vi "FGV_Id_Iq_ES.vi"(6 "Buffer Size":i32=10000, 7 "Command":T1, 8 "error in (no error)":errorcluster, 10 "Iq":sgl, 11 "Id":sgl) -> (0 "error out":errorcluster, 3 "Buffer":sgl[][](array[numeric]), 5 "Buffer Index":i32)   [LabVIEW 2015]
uses:
  Data_Queue_Command.ctl
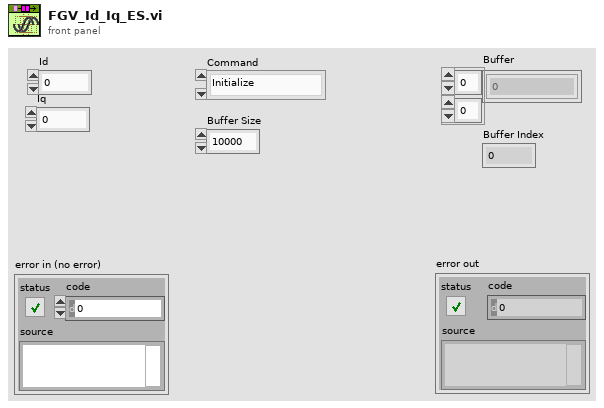
[diagram p1: front panel]
types:
  T1 = typedef "Data_Queue_Command.ctl" = enum16{"Initialize", "Write Sample", "Pull Array", "Close"}
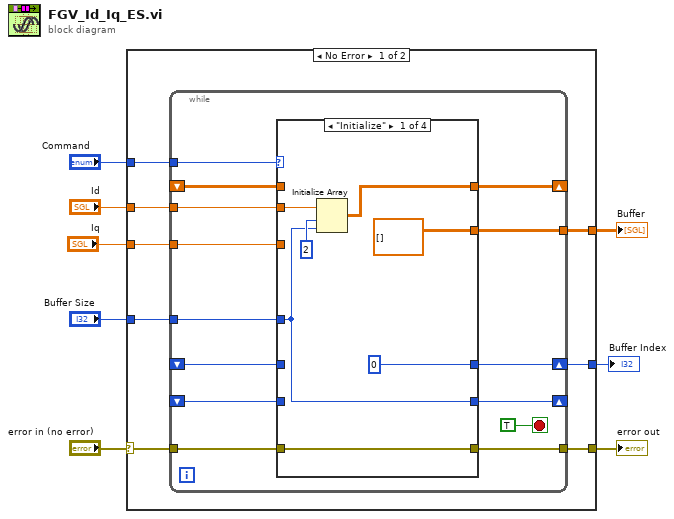
[diagram p0: block diagram]
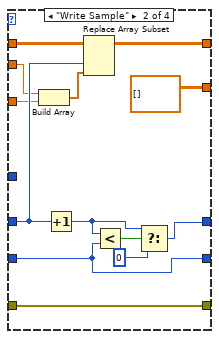
[diagram p2: hidden frame]
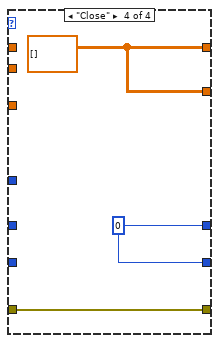
[diagram p4: hidden frame]
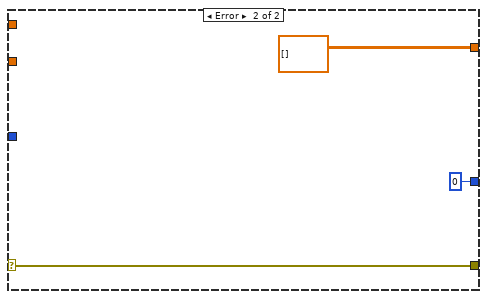
[diagram p5: hidden frame]
diagram:
  n1 = case shown="No Error" "error in (no error)" {
    selector: "error in (no error)" -> [w12 w60]
    tunnel: [w11 w60] -> w7
    tunnel: "Command" -> [w16 _]
    tunnel: "Buffer Size" -> [w15 _]
    tunnel: "Id" -> [w14 _]
    tunnel: [w13 sgl[][] []] -> w3
    tunnel: "Iq" -> [w10 _]
    tunnel: [w9 0 ("f")] -> w1
    frame No Error {
      n2 = while {
        tunnel: w16 -> [w29]
        tunnel: w15 -> [w28]
        tunnel: w14 -> [w27]
        shift-right: [w26] -> _
        shift-left: _ -> [w25]
        shift-right: [w24] -> _
        shift-left: _ -> [w23]
        shift-right: [w22] -> w9
        shift-left: _ -> [w21]
        tunnel: [w20] -> w13
        tunnel: w12 -> [w19]
        tunnel: [w18] -> w11
        tunnel: w10 -> [w17]
        stop <- TRUE stop-if-true
        n3 = case shown="\"Initialize\"" w29 {
          tunnel: w28 -> [w31 _ _ _]
          tunnel: w27 -> [w37 w40 _ _]
          tunnel: [w36 w45 w52 w57] -> w26
          tunnel: w25 -> [_ w50 w52 _]
          tunnel: [w31 w44 w53 w56] -> w24
          tunnel: w23 -> [_ w44 w53 _]
          tunnel: [0 ("Buffer Index") w46 w54 w56] -> w22
          tunnel: w21 -> [_ w41 w54 _]
          tunnel: [sgl[][] [] sgl[][] [] w52 w57] -> w20
          tunnel: w19 -> [w33 w42 w51 w55]
          tunnel: [w33 w42 w51 w55] -> w18
          tunnel: w17 -> [_ w39 _ _]
          frame "Initialize" {
            n4 = Initialize Array(w37, 2 ("dimension size"), w31) -> (w36:sgl[][])
          }
          frame "Write Sample" {
            n5 = Build Array(w40, w39) -> (w38:sgl[])
            n6 = Increment(x=w41) -> (x+1=w48:i32)
            n7 = Replace Array Subset(array=w50, new element=w38, index (col)=w41) -> (w45:sgl[][])  [unwired: 1 in]
            n8 = Less?(x=w48, y=w44) -> (x < y?=w49:bool)
            n9 = Select(t=w48, s=w49, f=0) -> (s? t:f=w46:i32)
          }
          frame "Pull Array" {
          }
          frame "Close" {
            w56 = 0 ("f")
            w57 = sgl[][] []
          }
        }
      }
    }
    frame Error {
    }
  }
  "Buffer" <- w3
  "error out" <- w7
  "Buffer Index" <- w1
